vi "Get Window Handle At Point.vi"(8 "error in (no error)":errorcluster, 11 "Point":T1) -> (0 "error out":errorcluster, 3 "hWnd":i32)   [LabVIEW 2019, in "Window.lvlib"]
doc: "Get the window handle of the window visible at the given point. Point is in screen coordinates."
uses:
  Window.lvlib
  User32.dll
  _2D/Point.ctl
  _2D/2D.lvlib
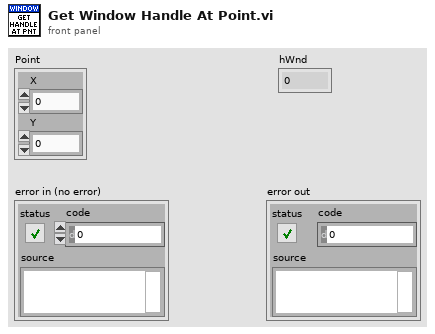
[diagram p1: front panel]
types:
  T1 = typedef "2D.lvlib/Point.ctl" = cluster{"X":i16, "Y":i16}
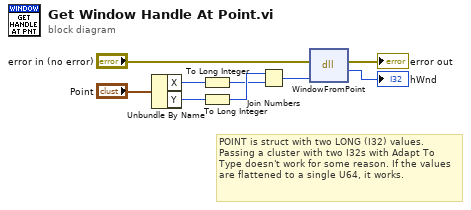
[diagram p0: block diagram]
diagram:
  # "POINT is struct with two LONG (I32) values.\nPassing a cluster with two I32s with Adapt To Type doesn't work for some reason. If the values are flattened to a single U64, it works."
  n1 = Unbundle By Name("Point") -> ("X"=w8:i16, "Y"=w7:i16)
  n2 = To Long Integer(number=w8) -> (32bit integer=w3:i32)
  n3 = To Long Integer(number=w7) -> (32bit integer=w4:i32)
  n4 = Join Numbers(hi=w4, lo=w3) -> ((hi.lo)=w6:u64)
  n5 = dll-call lib="user32.dll" fn="WindowFromPoint"(error in="error in (no error)", "point"=w6) -> (error out=→"error out":errorcluster, "hWnd"=→"hWnd":i32)  [unwired: 2 in, 2 out]
